vi "Alazar_SetRecord.vi"(9 "Pts to Acquire":u32, 10 "Records":u32=1, 11 "DeviceIn":i32) -> (0 "Return Code":u32, 2 "RecordOut":T1={"Count"=1, "Presize"=1, "Length"=0}, 3 "DeviceOut":i32)   [LabVIEW 2022 SP3]
doc: "_____AlazarTech, Scope_____\n\nConfigure the number of records for the device to capture."
uses:
  Record.ctl
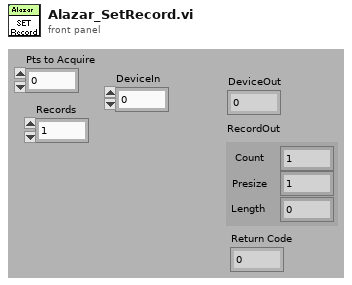
[diagram p1: front panel]
types:
  T1 = typedef "Record.ctl" = cluster{"Count":u32, "Presize":u32, "Length":u32}
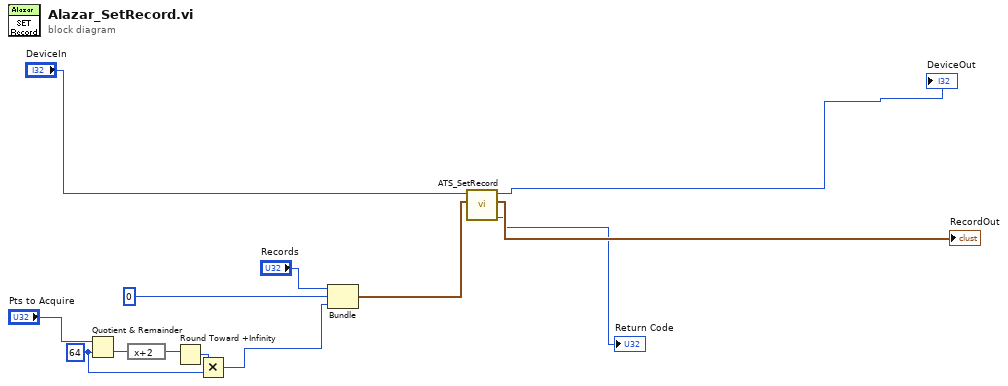
[diagram p0: block diagram]
diagram:
  w8 = u32 64 ("y")
  n1 = Quotient & Remainder(x="Pts to Acquire", y=w8) -> (floor(x/y)=w6:u32)  [unwired: 1 out]
  n2 = expression code="x+2"(w6) -> (w5:u32)
  n3 = Round Toward +Infinity(x=w5) -> (ceil(x): smallest int >= x=w7:u32)
  n4 = Multiply(x=w7, y=w8) -> (x*y=w1:u32)
  n5 = Bundle("Records"="Records", "Count"=u32 0, w1) -> (w3:cluster{"Records":u32, "Count":u32, u32})  [unwired: 1 in]
  n6 = call "ATS_SetRecord.vi"("RecordIn"=w3, "DeviceIn"="DeviceIn") -> ("Return Code"=→"Return Code":u32, "RecordOut"=→"RecordOut":T1, "DeviceOut"=→"DeviceOut":i32)  [unwired: 7 in]
